vi "Da rif freq a rif RPM.vi"(11 "Riferimento Frequenza":dbl) -> (3 "Riferimento RPM":dbl)   [LabVIEW 2019]
uses:
  Global config keb.vi
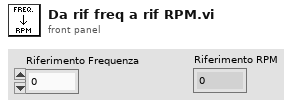
[diagram p1: front panel]
types:
  T1 = typedef "ConfigurazioneKeb.ctl" = cluster{"Freq nom":dbl, "RPM nom":dbl, "Pot nom":dbl, "I nom":dbl, "V nom":dbl, "Rpm max":dbl, "Tipo Motore":dbl}
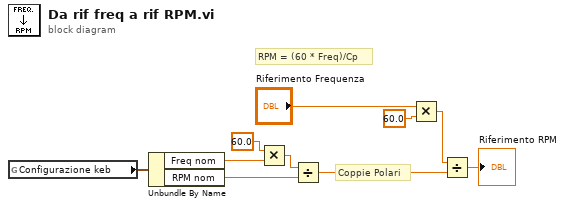
[diagram p0: block diagram]
diagram:
  # "Coppie Polari"
  # "RPM = (60 * Freq)/Cp"
  n1 = global read "Global config keb.vi" "Configurazione keb"() -> (w10:T1)
  n2 = Unbundle By Name(w10) -> ("Freq nom"=w7:dbl, "RPM nom"=w5:dbl)
  n3 = Multiply(x=60.0, y=w7) -> (x*y=w6:dbl)
  n4 = Divide(x=w6, y=w5) -> (x/y=w2:dbl)
  n5 = Multiply(x="Riferimento Frequenza", y=60.0) -> (x*y=w3:dbl)
  n6 = Divide(x=w3, y=w2) -> (x/y=→"Riferimento RPM":dbl)
